vi "control_select.vi"() -> ()   [LabVIEW 2014]
panel:
  out "数值":i32
  in  "选项卡控件":enum32{"s 1", "s23"}(tab)
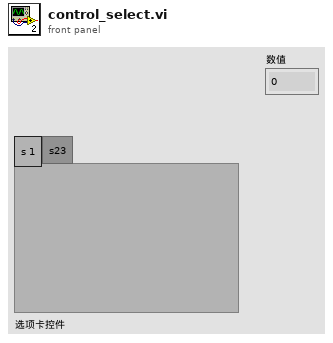
[diagram p1: front panel]
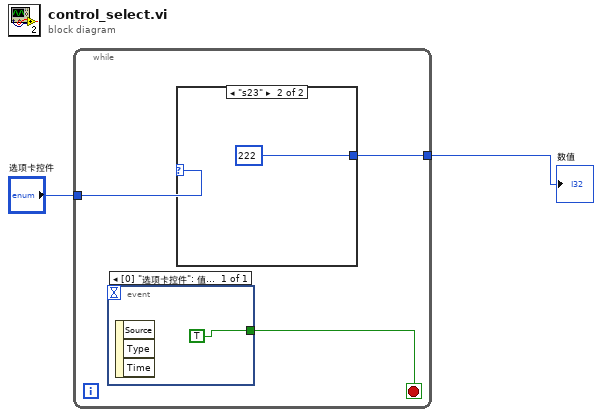
[diagram p0: block diagram]
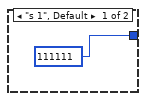
[diagram p2: hidden frame]
diagram:
  n1 = while {
    tunnel: "选项卡控件" -> [w5]
    tunnel: [w3] -> w1
    stop <- w4 stop-if-true
    n2 = event shown="[0] \"选项卡控件\": 值改变" {
      selector: _ -> [_]
      dyn-events: _ -> [_]
      timeout: _ -> [_]
      tunnel: [TRUE] -> w4
      event "选项卡控件": Value Change {
        n3 = event-data() -> ()  [unwired: 1 in, 3 out]
      }
    }
    n4 = case shown="\"s23\"" w5 {
      tunnel: [111111 222] -> w3
      frame "s 1", Default {
      }
      frame "s23" {
      }
    }
  }
  "数值" <- w1
